vi "LV to ITX  Retrieve Equation.vi"(0 "File or Folder Path":path, 1 "Data Type":T2, 2 "DAT header length":i32=11, 5 "offset":i32, 7 "length":i32=1, 9 "index":T3={"a"=4, "b"=10, "c"=7, "d"=9, "f"=2, "N1"=2, "N2"=0, "N3"=0, "N4"=0, "g"=1}, 11 "formula (parameters: a,b,c,d,f,g). g = x":string="y1 = g;\ny2 = b;", 12 "Enum 2":T1, 13 "data index":i32, 14 "data length":i32=500) -> (4 "y1 vs g":cluster{dbl[], dbl[]}[](graph), 6 "y2 vs g":cluster{dbl[], dbl[]}[](graph), 8 "2D":dbl[][](graph), 10 "N":T4={"N1"=73.16571153186332, "N2"=3605738918.935894, "N3"=3605738918.935894, "N4"=3605738918.935894} {"N4" format="%#_6p"; "N3" format="%#_6p"; "N2" format="%#_6p"; "N1" format="%#_6p"}, 15 "Comments":string)   [LabVIEW 2016, in "Data.ITX.lvclass"]
uses:
  Data.ITX.lvclass
  <userlib>/LevyLab/Graph Utilities/graph_utilities.lvclass
  <vilib>/gmath/NI_Gmath.lvlib
  Data.DAT/Data.DAT.lvclass
  Data.TDMS/Data.TDMS.lvclass
  C:/user/patrick/git/LV-to-ITX/src/Data/Data.lvclass
  <vilib>/Utility/miscctls.llb/LVOffsetAndMultiplierTypeDef.ctl
  Typedefs/Retrieve Index.ctl
  Typedefs/Retrieve N Results.ctl
  Typedefs/Retrieve Data Type.ctl
  Typedefs/Retrieve Formula Type.ctl
panel:
  in  "2D graph:\non = y1\noff = y2":bool=TRUE
  in  "D  is time?":bool
  in  "B is time?":bool
  out "time":string[][](table)
  in  "Use Folder Index File?":bool
  in  "Generate Folder Index File?":bool
  in  "Ez name":string="Ez name"
  in  "Ey name":string="Ey name"
  in  "Ex name":string="Ex name"
  in  "C y name":string="C y name"
  in  "D x name":string="D x name"
  in  "A y name":string="A y name"
  in  "B x name":string="B x name"
  out "Index, Wavenames":string[][](table)
  in  "recolor traces?":bool=TRUE
  in  "Ex":T5={"Offset"=0.0, "Multiplier"=1.0}
  in  "Ey":T5={"Offset"=0.0, "Multiplier"=1.0}
  out "Path":path
  out "counter":i32=9
  out "pattern":string="*.itx"
  # "YOU CAN CHOOSE THE FORMULA TYPE:"
  # "EQUATION"
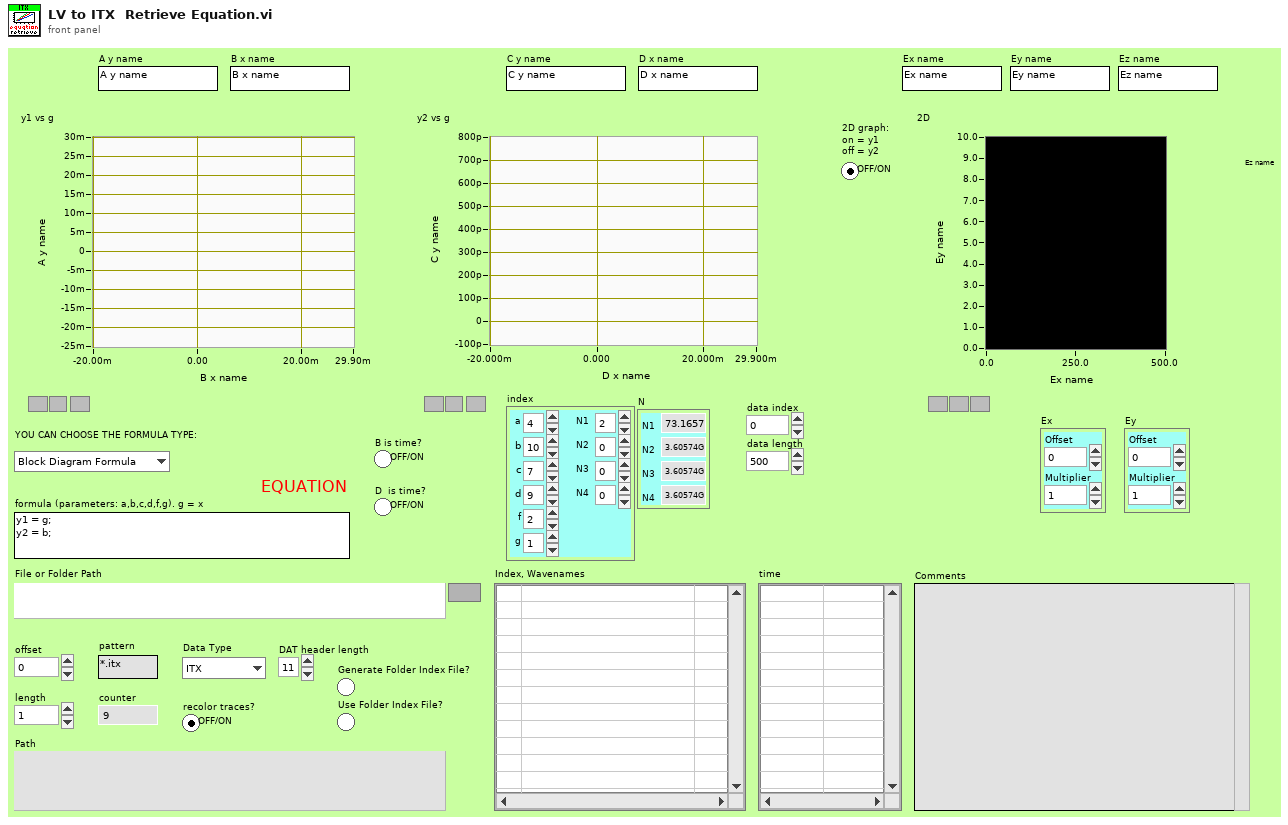
[diagram p1: front panel]
types:
  T1 = typedef "Data.ITX.lvclass/Retrieve Formula Type.ctl" = enum16{"Block Diagram Formula", "String Formula"}
  T2 = typedef "Data.ITX.lvclass/Retrieve Data Type.ctl" = enum16{"ITX", "ITX w/ 2D", "DAT", "TDMS"}
  T3 = typedef "Data.ITX.lvclass/Retrieve Index.ctl" = cluster{"a":i32, "b":i32, "c":i32, "d":i32, "f":i32, "N1":i32, "N2":i32, "N3":i32, "N4":i32, "g":i32}
  T4 = typedef "Data.ITX.lvclass/Retrieve N Results.ctl" = cluster{"N1":dbl, "N2":dbl, "N3":dbl, "N4":dbl}
  T5 = typedef "LVOffsetAndMultiplierTypeDef.ctl" = cluster{"Offset":dbl, "Multiplier":dbl}
  T6 = typedef "Data.lvclass/Dictionary--cluster.ctl" = cluster{"key":string, "value":variant}
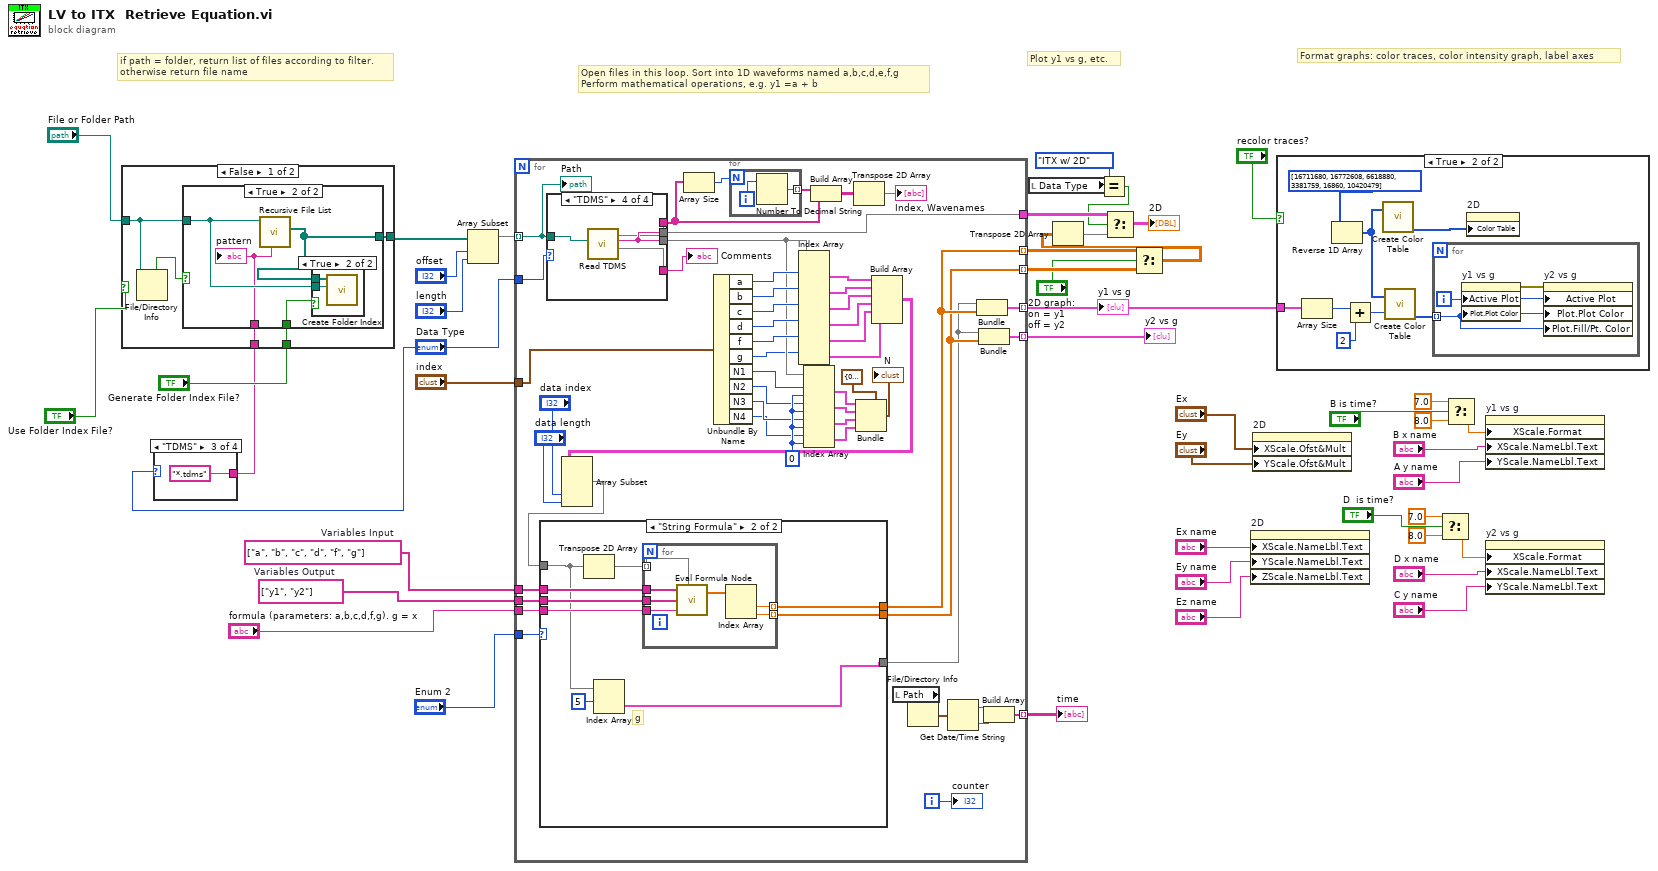
[diagram p0: block diagram]
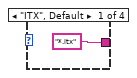
[diagram p2: hidden frame]
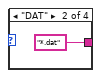
[diagram p3: hidden frame]
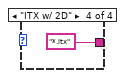
[diagram p4: hidden frame]
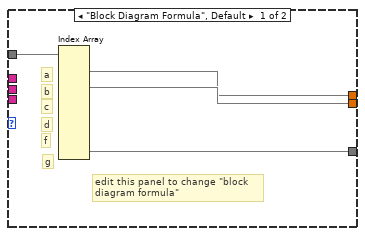
[diagram p6: hidden frame]
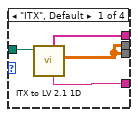
[diagram p7: hidden frame]
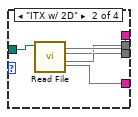
[diagram p8: hidden frame]
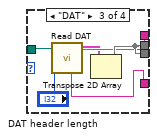
[diagram p9: hidden frame]
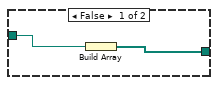
[diagram p10: hidden frame]
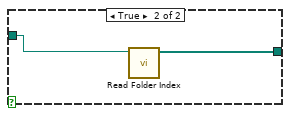
[diagram p12: hidden frame]
diagram:
  w10 = string[] ["a", "b", "c", "d", "f", "g"]  # Variables Input
  w3 = string[] ["y1", "y2"]  # Variables Output
  # "Plot y1 vs g, etc."
  # "Format graphs: color traces, color intensity graph, label axes"
  # "Open files in this loop. Sort into 1D waveforms named a,b,c,d,e,f,g\nPerform mathematical operations, e.g. y1 =a + b"
  # "if path = folder, return list of files according to filter.\notherwise return file name"
  n1 = case shown="\"TDMS\"" "Data Type" {
    tunnel: ["*.itx" ("pattern") "*.dat" ("pattern") "*.tdms" ("pattern") "*.itx" ("pattern")] -> w2
    frame "ITX", Default {
    }
    frame "DAT" {
    }
    frame "TDMS" {
    }
    frame "ITX w/ 2D" {
    }
  }
  n2 = case shown="False" "Use Folder Index File?" {
    tunnel: [w52 w63] -> w43
    tunnel: "File or Folder Path" -> [w54 w64]
    tunnel: "Generate Folder Index File?" -> [w51 _]
    tunnel: w2 -> [w50 _]
    frame False {
      n3 = File/Directory Info(path=w54) -> (directory=w53:bool)  [unwired: 1 in, 6 out]
      n4 = case shown="True" w53 {
        tunnel: [w56 w60] -> w52
        tunnel: w54 -> [w55 w59]
        tunnel: w51 -> [_ w58]
        tunnel: w50 -> [_ w57]
        frame False {
          n5 = Build Array(w55) -> (w56:path[])
        }
        frame True {
          n6 = call <vilib>:"Recursive File List.vi"("pattern"=w57, "Folder Path"=w59) -> ("All Files in Dir"=w60:path[])  [unwired: 5 in, 4 out]
          n7 = case shown="True" w58 {
            tunnel: w60 -> [_ w62]
            tunnel: w59 -> [_ w61]
            frame False {
            }
            frame True {
              n8 = call "Create Folder Index.vi"("File or Folder Path"=w61, "All Files in Dir"=w62) -> ()  [unwired: 9 in, 1 out]
            }
          }
          "pattern" <- w57
        }
      }
    }
    frame True {
      n9 = call "Read Folder Index.vi"("File or Folder Path"=w64) -> ("Files"=w63:path[])  [unwired: 9 in, 1 out]
    }
  }
  n10 = Array Subset(array=w43, index="offset", length="length") -> (w24:path[])
  n11 = for {
    tunnel: w24 -> [w115] mode=indexing
    tunnel: [w115] -> _ mode=indexing
    tunnel: [w114] -> w12 mode=indexing
    tunnel: [w113] -> w35 mode=indexing
    tunnel: [w108] -> w37
    tunnel: [w98] -> w27 mode=indexing
    tunnel: "formula (parameters: a,b,c,d,f,g). g = x" -> [w92]
    tunnel: w3 -> [w91]
    tunnel: w10 -> [w90]
    tunnel: "Data Type" -> [w89]
    tunnel: "index" -> [w70]
    tunnel: "Enum 2" -> [w88]
    tunnel: [w82] -> w8 mode=indexing
    tunnel: [w81] -> w6 mode=indexing
    i -> [w117]
    w107 = 0 ("disabled index (col)")
    n12 = case shown="\"TDMS\"" w89 {
      tunnel: [w141 w147 w152 w157] -> w116
      tunnel: [w142 w145 w153 w156] -> w69
      tunnel: w115 -> [w143 w148 w154 w158]
      tunnel: [w140 w146 w151 w155] -> w109
      tunnel: [w142 w144 w153 w156] -> w108
      frame "ITX", Default {
        n13 = call "ITX to LV 2.1 1D.vi"("file (use dialog)"=w143) -> ("1D arrays"=w142:dbl[][], "Notes"=w141:string, "base wavenames"=w140:string[])  [unwired: 5 in, 3 out]
      }
      frame "ITX w/ 2D" {
        n14 = call-dynamic "Read File.vi"("ITX"=w148) -> (1:w145, 2:w144, 4:w147, 5:w146)  [unwired: 5 in, 2 out]
      }
      frame "DAT" {
        n15 = call "Read DAT.vi"(10:"DAT header length", 11:w154) -> ("Data (Dictionary)"=w150:T6[], "Notes"=w152:string, 5:w151)  [unwired: 6 in, 1 out]
        n16 = Transpose 2D Array(2D array=w150) -> (transposed array=w153:T6[][])
      }
      frame "TDMS" {
        n17 = call "Read TDMS.vi"(10:w158) -> ("Notes"=w156:string, 4:w157, 5:w155)  [unwired: 5 in, 3 out]
      }
    }
    "Comments" <- w116
    n18 = Array Size(array=w109) -> (size(s)=w65:i32)
    n19 = Unbundle By Name(w70) -> ("a"=w106:i32, "b"=w105:i32, "c"=w104:i32, "d"=w103:i32, "f"=w93:i32, "g"=w68:i32, "N1"=w74:i32, "N2"=w73:i32, "N3"=w72:i32, "N4"=w71:i32)
    n20 = for {
      N: w65 -> [_]
      tunnel: [w138] -> w112 mode=indexing
      i -> [w139]
      n21 = Number To Decimal String(number=w139) -> (decimal integer string=w138:string)  [unwired: 1 in]
    }
    n22 = Index Array(array=w69, index (row) #1=w106, index (row) #2=w105, index (row) #3=w104, index (row) #4=w103, index (row) #5=w93, index (row) #6=w68) -> (element #1=w75:T6[], element #2=w76:T6[], element #3=w77:T6[], element #4=w78:T6[], element #5=w84:T6[], element #6=w67:T6[])  [unwired: 6 in]
    n23 = Index Array(array=w69, index (row) #1=w74, index (col) #1=w107, index (row) #2=w73, index (col) #2=w107, index (row) #3=w72, index (col) #3=w107, index (row) #4=w71, index (col) #4=w107) -> (element #1=w97:T6, element #2=w96:T6, element #3=w95:T6, element #4=w94:T6)
    n24 = Build Array(w112, w109) -> (w110:string[][])
    n25 = Transpose 2D Array(2D array=w110) -> (transposed array=→"Index, Wavenames":string[][])
    n26 = Bundle(cluster=cluster{"N1":dbl, "N2":dbl, "N3":dbl, "N4":dbl} {"N1"=0.0, "N2"=0.0, "N3"=0.0, "N4"=0.0}, "N1"=w97, "N2"=w96, "N3"=w95, "N4"=w94) -> (→"N":cluster{"N1":dbl, "N2":dbl, "N3":dbl, "N4":dbl})
    n27 = Build Array(w75, w76, w77, w78, w84, w67) -> (w80:T6[][])
    n28 = Array Subset(array=w80, index (col)="data index", length (col)="data length") -> (w83:T6[][])  [unwired: 2 in]
    n29 = case shown="\"String Formula\"" w88 {
      tunnel: [w120 w130] -> w81
      tunnel: w83 -> [w121 w124]
      tunnel: [w119 w129] -> w82
      tunnel: w92 -> [_ w128]
      tunnel: w91 -> [_ w127]
      tunnel: w90 -> [_ w126]
      tunnel: [w118 w122] -> w66
      frame "Block Diagram Formula", Default {
        # "g"
        # "f"
        # "d"
        # "c"
        # "b"
        # "a"
        # "edit this panel to change \"block\ndiagram formula\""
        n30 = Index Array(array=w121) -> (element #1=w119:T6[], element #2=w120:T6[], element #6=w118:T6[])  [unwired: 12 in, 3 out]
      }
      frame "String Formula" {
        # "g"
        n31 = Transpose 2D Array(2D array=w124) -> (transposed array=w125:T6[][])
        n32 = Index Array(array=w124, index (row)=5) -> (element=w122:T6[])  [unwired: 1 in]
        n33 = for {
          tunnel: w126 -> [w137]
          tunnel: w127 -> [w136]
          tunnel: w128 -> [w135]
          tunnel: w125 -> [w131] mode=indexing
          tunnel: [w133] -> w130 mode=indexing
          tunnel: [w132] -> w129 mode=indexing
          n34 = call <vilib>:"Eval Formula Node.vi"("Variables Input"=w137, "Input Values"=w131, "Variables Output"=w136, "formula"=w135) -> ("Output Values"=w134:dbl[])  [unwired: 1 in, 1 out]
          n35 = Index Array(array=w134) -> (element #1=w132:dbl, element #2=w133:dbl)  [unwired: 2 in]
        }
      }
    }
    n36 = local read "Path"() -> (w102:path)
    n37 = File/Directory Info(path=w102) -> (last mod=w101:timestamp)  [unwired: 1 in, 6 out]
    n38 = Get Date/Time String(seconds (now)=w101) -> (date string=w100:string, time string=w99:string)  [unwired: 2 in]
    n39 = Bundle(w66, w82) -> (w114:cluster{T6[], dbl[]})  [unwired: 1 in]
    n40 = Bundle(w66, w81) -> (w113:cluster{T6[], dbl[]})  [unwired: 1 in]
    n41 = Build Array(w100, w99) -> (w98:string[])
    "counter" <- w117
    "Path" <- w115
  }
  "y1 vs g" <- w12
  "y2 vs g" <- w35
  "time" <- w27
  n42 = local read "Data Type"() -> (w14:T2)
  n43 = Equal?(x=enum16{"ITX", "ITX w/ 2D", "DAT"}."ITX w/ 2D" ("Enum"), y=w14) -> (x = y?=w13:bool)
  n44 = Select(t=w8, s="2D graph:\non = y1\noff = y2", f=w6) -> (s? t:f=w7:dbl[][])
  n45 = Transpose 2D Array(2D array=w7) -> (transposed array=w39:dbl[][])
  n46 = Select(t=w37, s=w13, f=w39) -> (s? t:f=→"2D":T6[][])
  n47 = property on="2D" class="IntGraph (strict)"("XScale.NameLbl.Text"="Ex name", "YScale.NameLbl.Text"="Ey name", "ZScale.NameLbl.Text"="Ez name") -> ()  [unwired: 2 in, 2 out]
  n48 = property on="2D" class="IntGraph (strict)"("XScale.Ofst&Mult"="Ex", "YScale.Ofst&Mult"="Ey") -> ()  [unwired: 2 in, 2 out]
  n49 = case shown="True" "recolor traces?" {
    tunnel: w12 -> [_ w161]
    frame False {
    }
    frame True {
      n50 = Array Size(array=w161) -> (size(s)=w162:i32)
      n51 = Reverse 1D Array(array=u32[] [16711680, 16772608, 6618880, 3381759, 16860, 10420479] ("color scale")) -> (reversed array=w160:u32[])
      n52 = Add(x=w162, y=2 ("x")) -> (x+y=w166:i32)
      n53 = call <userlib>:"Create Color Table.vi"("Colors []"=w160) -> ("Color Tbl"=w164:u32[])  [unwired: 1 in, 3 out]
      n54 = call <userlib>:"Create Color Table.vi"("Colors []"=w160, "Size (256)"=w166) -> ("Color Tbl"=w163:u32[])  [unwired: 3 out]
      n55 = for {
        tunnel: w163 -> [w167] mode=indexing
        i -> [w168]
        n56 = property on="y1 vs g" class="XYGraph (strict)"("Active Plot"=w168, "Plot.Plot Color"=w167) -> (error out=w169:errorcluster)  [unwired: 2 in, 1 out]
        n57 = property on="y2 vs g" class="XYGraph (strict)"(error in=w169, "Active Plot"=w168, "Plot.Plot Color"=w167, "Plot.Fill/Pt. Color"=w167) -> ()  [unwired: 1 in, 2 out]
      }
      n58 = property on="2D" class="IntGraph (strict)"("Color Table"=w164) -> ()  [unwired: 2 in, 2 out]
    }
  }
  n59 = Select(t=7.0, s="D  is time?", f=8.0) -> (s? t:f=w20:dbl)
  n60 = Select(t=7.0, s="B is time?", f=8.0) -> (s? t:f=w21:dbl)
  n61 = property on="y1 vs g" class="XYGraph (strict)"("XScale.Format"=w21, "XScale.NameLbl.Text"="B x name", "YScale.NameLbl.Text"="A y name") -> ()  [unwired: 2 in, 2 out]
  n62 = property on="y2 vs g" class="XYGraph (strict)"("XScale.Format"=w20, "XScale.NameLbl.Text"="D x name", "YScale.NameLbl.Text"="C y name") -> ()  [unwired: 2 in, 2 out]
